vi "GeneralPIDMaintain.vi"(4 "PID gains":T1={"proportional gain (Kc)"=1.0, "integral time (Ti, min)"=0.01, "derivative time (Td, min)"=0.0} {"derivative time (Td, min)" format="%.3f"; "integral time (Ti, min)" format="%.3f"; "proportional gain (Kc)" format="%.3f"}, 6 "Output Range":cluster{"output high":dbl, "output low":dbl}={"output high"=100.0, "output low"=-100.0} {"output low" format="%.2f"; "output high" format="%.2f"}, 7 "Initialize":bool, 8 "Lower Power Limit":dbl format="%#_13g", 9 "Upper Power Limit":dbl format="%#_13g", 10 "Power":dbl format="%#_13g", 11 "Encoder Position":i32) -> (2 "Power Out":dbl)   [LabVIEW 2018]
uses:
  <vilib>/addons/control/pid/pid.llb/PID (DBL).vi
  <vilib>/addons/control/pid/NI_PID_pid.lvlib
panel:
  in  "Hold Position":i32
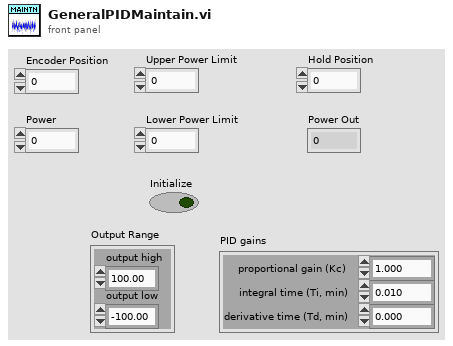
[diagram p1: front panel]
types:
  T1 = cluster{"proportional gain (Kc)":dbl, "integral time (Ti, min)":dbl, "derivative time (Td, min)":dbl}
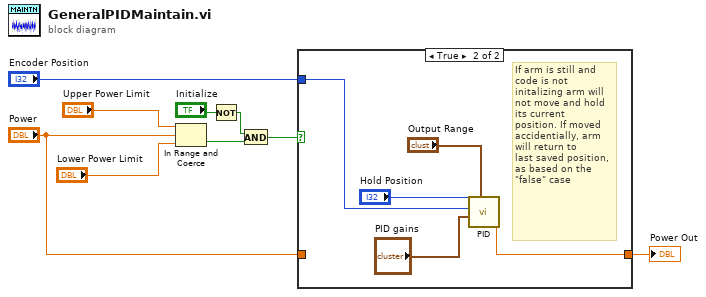
[diagram p0: block diagram]
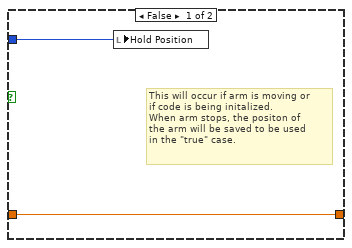
[diagram p2: hidden frame]
diagram:
  n1 = In Range and Coerce(upper limit="Upper Power Limit", x="Power", lower limit="Lower Power Limit") -> (In Range?=w4:bool)  [unwired: 1 out]
  n2 = Not(x="Initialize") -> (.not. x?=w2:bool)
  n3 = And(x=w2, y=w4) -> (x .and. y?=w3:bool)
  n4 = case shown="True" w3 {
    tunnel: "Encoder Position" -> [w10 w16]
    tunnel: [w11 w13] -> w6
    tunnel: "Power" -> [w11 _]
    frame False {
      # "This will occur if arm is moving or \nif code is being initalized.\nWhen arm stops, the positon of\nthe arm will be saved to be used\nin the \"true\" case."
      n5 = local write "Hold Position"(w10) -> ()
    }
    frame True {
      # "If arm is still and\ncode is not initalizing arm will not move and hold its current\nposition. If moved\naccidentially, arm \nwill return to \nlast saved position,\nas based on the \n\"false\" case"
      n6 = call-poly <vilib>:"PID.vi"("output range"="Output Range", "PID gains"="PID gains", "process variable"=w16, "setpoint"="Hold Position") -> ("output"=w13:dbl)  [unwired: 6 in, 1 out]
    }
  }
  "Power Out" <- w6
